vi "TSET-Advanced CSM Search.vi"() -> ()   [LabVIEW 2017]
uses:
  src/user.lib/_NEVSTOP/Communicable State Machine(CSM)/_tool/_Support/csm-tool-support.lvlib
panel:
  out "Is CSM Module?":bool
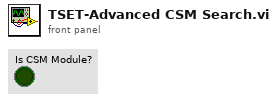
[diagram p1: front panel]
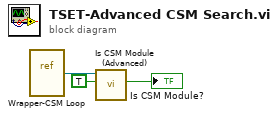
[diagram p0: block diagram]
diagram:
  n1 = vi-ref "Wrapper-CSM Loop.vi"() -> (w2:refnum<vi>)
  n2 = call "Is CSM Module (Advanced).vi"("Active(F)"=TRUE, "VIRef"=w2) -> ("Is CSM Module?"=→"Is CSM Module?":bool)  [unwired: 7 in, 2 out]
